vi "validate_arguments.vi"(6 "vmin":refnum<vi>, 9 "upper time":refnum<vi>, 10 "lower time":refnum<vi>, 11 "vmax":refnum<vi>) -> (3 "Problem":bool, 4 "String":string)   [LabVIEW 2015]
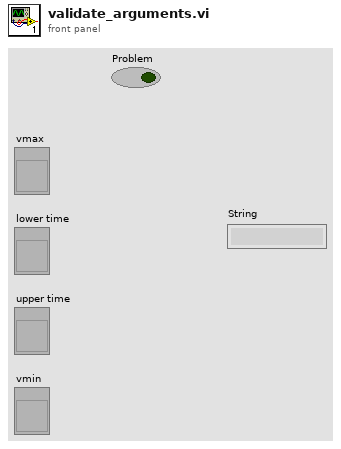
[diagram p1: front panel]
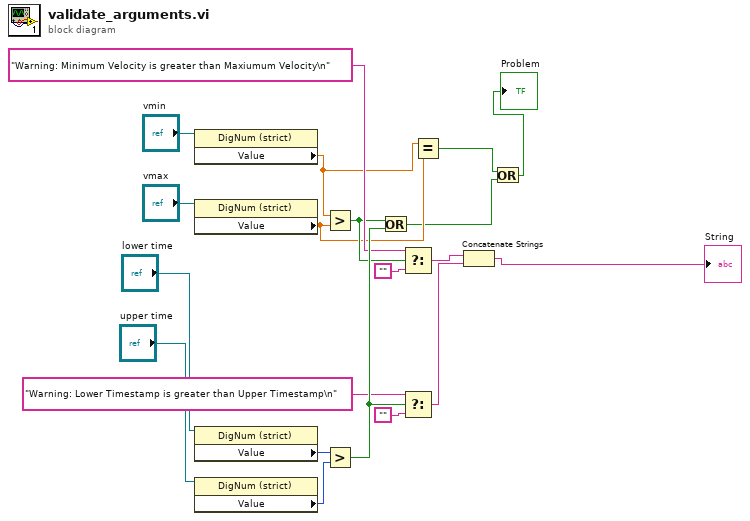
[diagram p0: block diagram]
diagram:
  n1 = property class="DigNum (strict)"(reference="vmin") -> ("Value"=w6:dbl)  [unwired: 1 in, 2 out]
  n2 = property class="DigNum (strict)"(reference="vmax") -> ("Value"=w5:dbl)  [unwired: 1 in, 2 out]
  n3 = property class="DigNum (strict)"(reference="lower time") -> ("Value"=w16:i64)  [unwired: 1 in, 2 out]
  n4 = property class="DigNum (strict)"(reference="upper time") -> ("Value"=w15:i64)  [unwired: 1 in, 2 out]
  n5 = Greater?(x=w6, y=w5) -> (0:w7:bool)
  n6 = Greater?(x=w16, y=w15) -> (0:w14:bool)
  n7 = Or(x=w7, y=w14) -> (x .or. y?=w3:bool)
  n8 = Select(t="Warning: Minimum Velocity is greater than Maxiumum Velocity\n", s=w7, f="") -> (s? t:f=w9:string)
  n9 = Select(t="Warning: Lower Timestamp is greater than Upper Timestamp\n", s=w14, f="") -> (s? t:f=w8:string)
  n10 = Equal?(x=w6, y=w5) -> (x = y?=w4:bool)
  n11 = Concatenate Strings(w9, w8) -> (→"String":string)
  n12 = Or(x=w4, y=w3) -> (x .or. y?=→"Problem":bool)
